vi "test Parse Device Info_1.vi"(11 "Test Case In":refnum<class "test Electronic Datasheet.lvclass">) -> (0 "error out":errorcluster, 3 "Test Case Out":refnum<class "test Electronic Datasheet.lvclass">)   [LabVIEW 2024, in "test Electronic Datasheet.lvclass"]
uses:
  test Electronic Datasheet.lvclass
  C:/Program Files/National Instruments/LabVIEW 2024/vi.lib/Astemes/LUnit/Test Case.lvclass
  <vilib>/PNR/JSONtext Object Serialization/Generic Object Serializer/Generic Object Serializer.lvclass
  C:/Program Files/National Instruments/LabVIEW 2024/vi.lib/JDP Science/JSONtext/LVClass Serializer/JSONtext LVClass Serializer.lvclass
  <vilib>/PNR/JSONtext Object Serialization/Generic Object Serializer/Type Name Handling.ctl
  <vilib>/PNR/JSONtext Object Serialization/Generic Object Serializer/Generic Object Serializer.lvclass/Generic Object Serializer.ctl
  <vilib>/Astemes/LUnit/Test Case.lvclass/Test Case.ctl
  99df47cb-525e-4171-a825-741cf93afc66.vi
  4993e8ee-a06a-463a-9684-69129f64d5ce.vi
  <vilib>/PNR/JSONtext Object Serialization/Generic Object Serializer/Write Type Name Handling.vi
  <vilib>/Astemes/LUnit/Append Pass Result.vi
  <vilib>/Astemes/LUnit/Append Fail Result.vi
  <vilib>/Astemes/LUnit/Describe Comparison.vi
  4993e8ee-a06a-463a-9684-69129f64d5ce.vi/9c5d11cd-9439-4240-a1ee-d9baace9c924.vi
  <vilib>/Astemes/LUnit/Run In UI.vi
  <vilib>/Utility/error.llb/Clear Errors.vi
  Electronic Datasheet/utils/Electronic Datasheet_GetAttributes.vi
  <vilib>/JDP Science/JSONtext/Variant to JSON Text.vi
  <vilib>/Astemes/LUnit/Describe Variant.vi
  Electronic Datasheet/Electronic Datasheet.lvclass
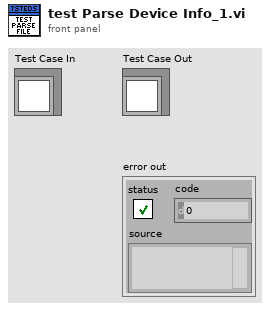
[diagram p1: front panel]
types:
  T1 = typedef "Generic Object Serializer.lvclass/Type Name Handling.ctl" = enum16{"None", "Inline"}
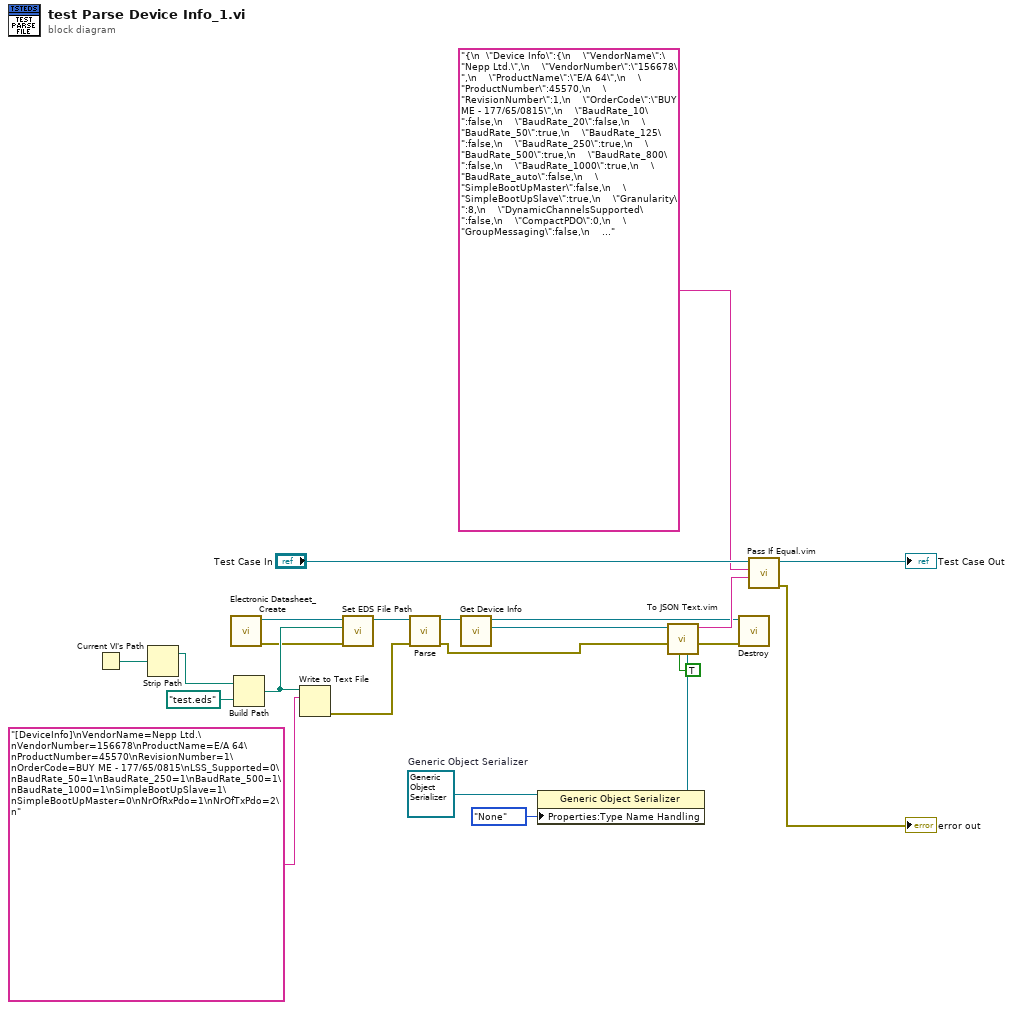
[diagram p0: block diagram]
diagram:
  w11 = refnum<class "Generic Object Serializer.lvclass"> refnum  # Generic Object Serializer
  n1 = Current VI's Path() -> (path=w19:path)
  n2 = Strip Path(path=w19) -> (stripped path=w18:path)  [unwired: 1 out]
  n3 = call "Electronic Datasheet_Create.vi"() -> ("Error Out"=w3:errorcluster, "reference out"=w4:refnum<class "Electronic Datasheet.lvclass">)  [unwired: 10 in]
  n4 = Build Path(base path=w18, name or relative path=path "test.eds") -> (appended path=w17:path)
  n5 = Write to Text File(file (use dialog)=w17, text="[DeviceInfo]\nVendorName=Nepp Ltd.\nVendorNumber=156678\nProductName=E/A 64\nProductNumber=45570\nRevisionNumber=1\nOrderCode=BUY ME - 177/65/0815\nLSS_Supported=0\nBaudRate_50=1\nBaudRate_250=1\nBaudRate_500=1\nBaudRate_1000=1\nSimpleBootUpSlave=1\nSimpleBootUpMaster=0\nNrOfRxPdo=1\nNrOfTxPdo=2\n") -> (error out=w15:errorcluster)  [unwired: 2 in, 2 out]
  n6 = call "Set EDS File Path.vi"("error in"=w3, "EDS File Path"=w17, "reference in"=w4) -> ("reference out"=w20:refnum<class "Electronic Datasheet.lvclass">)  [unwired: 7 in, 1 out]
  n7 = call "Parse.vi"("error in"=w15, "reference in"=w20) -> ("error out"=w8:errorcluster, "reference out"=w13:refnum<class "Electronic Datasheet.lvclass">)  [unwired: 8 in]
  n8 = call "Get Device Info.vi"("reference in"=w13) -> ("Device Info"=w7:refnum<class "Device Info.lvclass">, "reference out"=w2:refnum<class "Electronic Datasheet.lvclass">)  [unwired: 8 in, 1 out]
  n9 = property class="Generic Object Serializer"(reference=w11, "Properties:Type Name Handling"=Type_Name_Handling."None" ("Type Name Handling")) -> (reference out=w10:refnum<class "Generic Object Serializer.lvclass">)  [unwired: 1 in, 1 out]
  n10 = call "To JSON Text.vim"("LVClass Serializer"=w10, "Pretty Print?"=TRUE, "error in (no error)"=w8, "Anything"=w7) -> ("error out"=w1:errorcluster, "<JSON>"=w5:string)  [unwired: 6 in]
  n11 = call-dynamic "Destroy.vi"("Error In"=w1, "reference in"=w2) -> ()  [unwired: 8 in, 2 out]
  n12 = call "Pass If Equal.vim"("Actual"=w5, "Expected"="{\n  \"Device Info\":{\n    \"VendorName\":\"Nepp Ltd.\",\n    \"VendorNumber\":\"156678\",\n    \"ProductName\":\"E/A 64\",\n    \"ProductNumber\":45570,\n    \"RevisionNumber\":1,\n    \"OrderCode\":\"BUY ME - 177/65/0815\",\n    \"BaudRate_10\":false,\n    \"BaudRate_20\":false,\n    \"BaudRate_50\":true,\n    \"BaudRate_125\":false,\n    \"BaudRate_250\":true,\n    \"BaudRate_500\":true,\n    \"BaudRate_800\":false,\n    \"BaudRate_1000\":true,\n    \"BaudRate_auto\":false,\n    \"SimpleBootUpMaster\":false,\n    \"SimpleBootUpSlave\":true,\n    \"Granularity\":8,\n    \"DynamicChannelsSupported\":false,\n    \"CompactPDO\":0,\n    \"GroupMessaging\":false,\n    \"NrOfRXPDO\":1,\n    \"NrOfTXPDO\":2,\n    \"LSS_Supported\":false,\n    \"LSS_Master\":false,\n    \"NG_Slave\":false,\n    \"NG_Master\":false,\n    \"NrOfNG_MonitoredNodes\":0\n  }\n}" ("<JSON>"), "LUnit Test Case In"="Test Case In") -> ("error out"=→"error out":errorcluster, "LUnit Test Case Out"=→"Test Case Out":refnum<class "test Electronic Datasheet.lvclass">)  [unwired: 7 in]
